vi "LvDataToMemory_PTR.vi"(8 "error in (no error)":errorcluster, 10 "Payload":variant, 11 "AddrQueueIn":refnum<queue>) -> (0 "error out":errorcluster, 1 "Supported Type?":bool, 2 "ByteArray":u8[](array[numeric]), 3 "AddrQueueOut":refnum<queue>)   [LabVIEW 2019, in "Memory Data Access.lvlib"]
uses:
  Memory Data Access.lvlib
  <vilib>/Utility/Data Type/Type Definitions/Data Type.ctl
  Global/Global.vi
  <vilib>/Utility/Data Type/NI_Data Type.lvlib
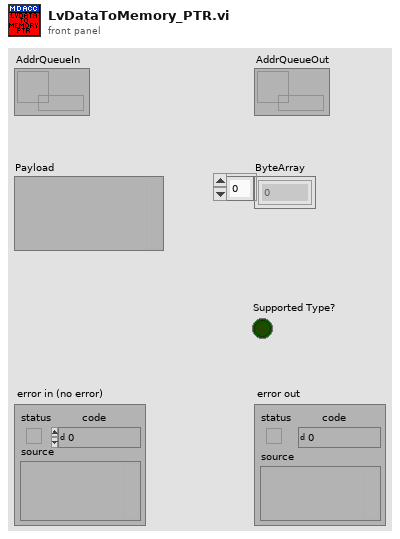
[diagram p1: front panel]
types:
  T1 = typedef "NI_Data Type.lvlib/Data Type.ctl" = enum8{"Invalid Type", "Void", "I8", "I16", "I32", "I64", "U8", "U16", "U32", "U64", "Single Float", "Double Float", "Extended Float", "Single Complex", "Double Complex", "Extended Complex", "Enum U8", "Enum U16", "Enum U32", "Enum U64", "Single Float With Unit", "Double Float With Unit", "Extended Float With Unit", "Single Complex with Unit", "Double Complex with Unit", "Extended Complex with Unit", "Boolean", "String", "Path", "Picture", "Tag", "Array", "Cluster", "Variant", "LV Variant", "Waveform", "Timestamp", "Digital Waveform", "Digital Data", "ExpressData", "Refnum", "External Data", "VI", "Poly VI", "LabVIEW Class Instance", "Fixed Point", "Set Collection", "Map Collection"}
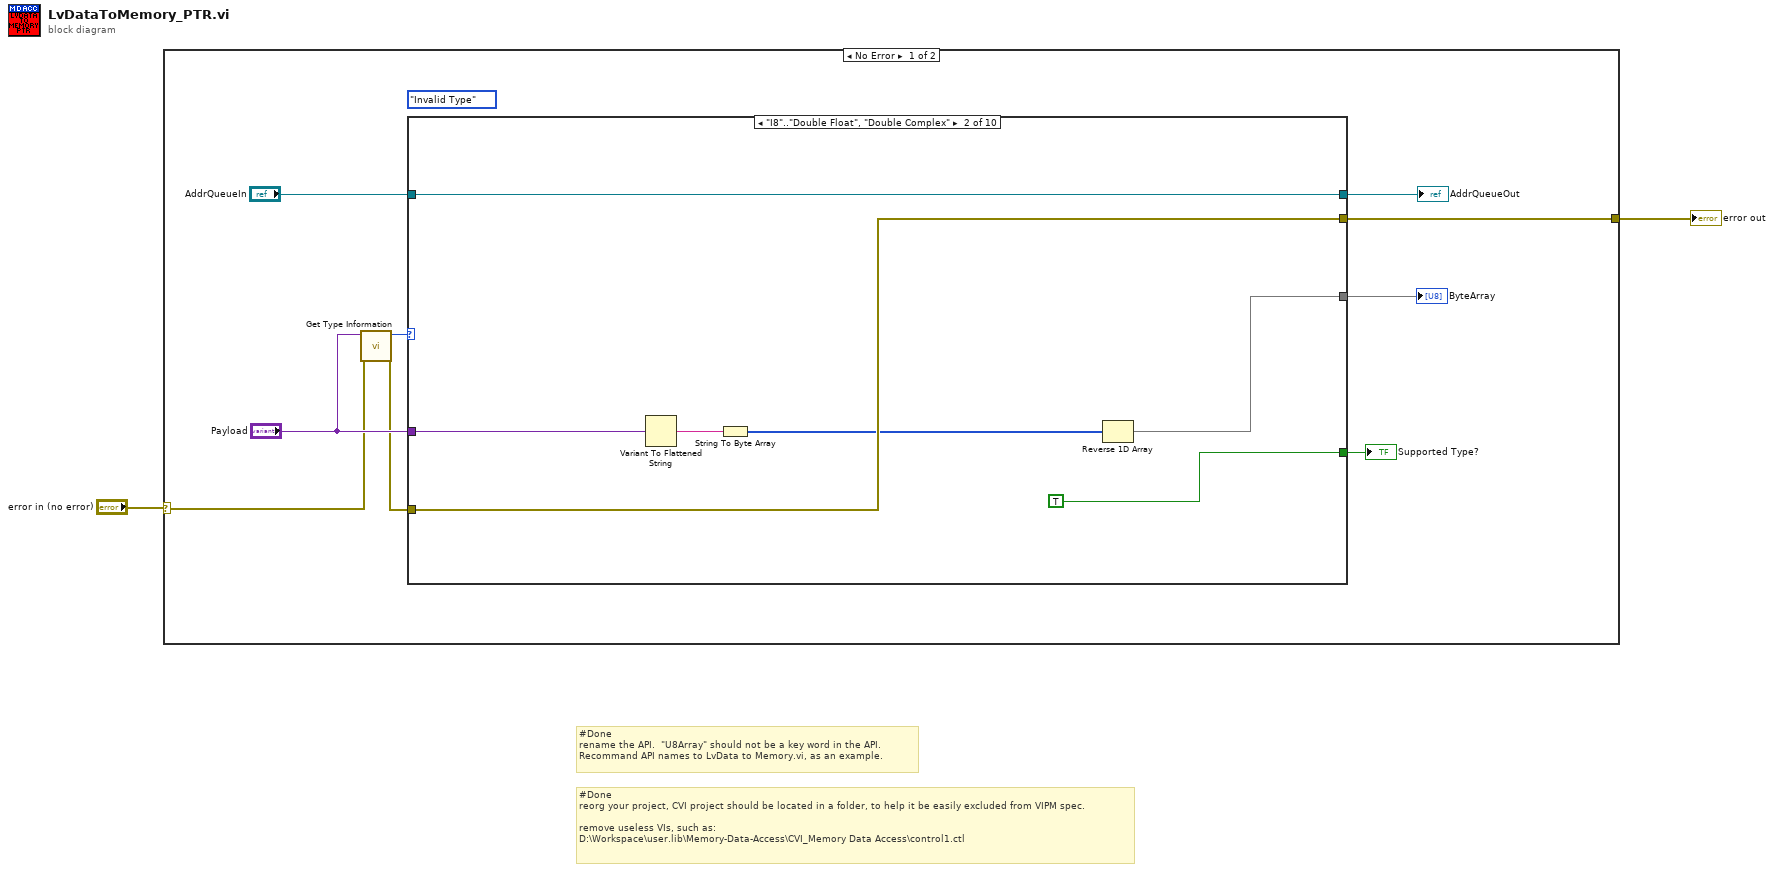
[diagram p0: block diagram]
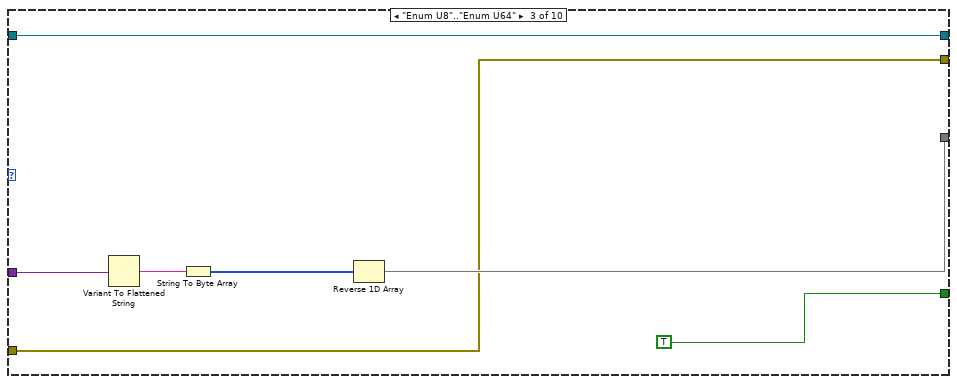
[diagram p3: hidden frame]
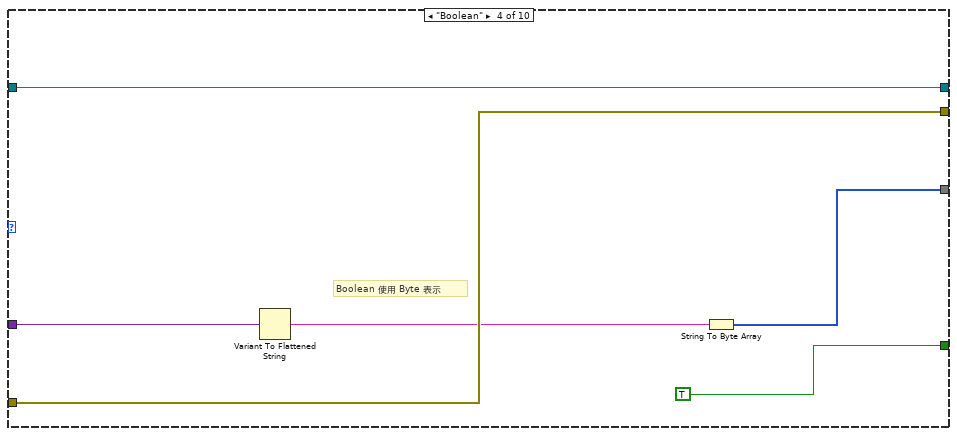
[diagram p4: hidden frame]
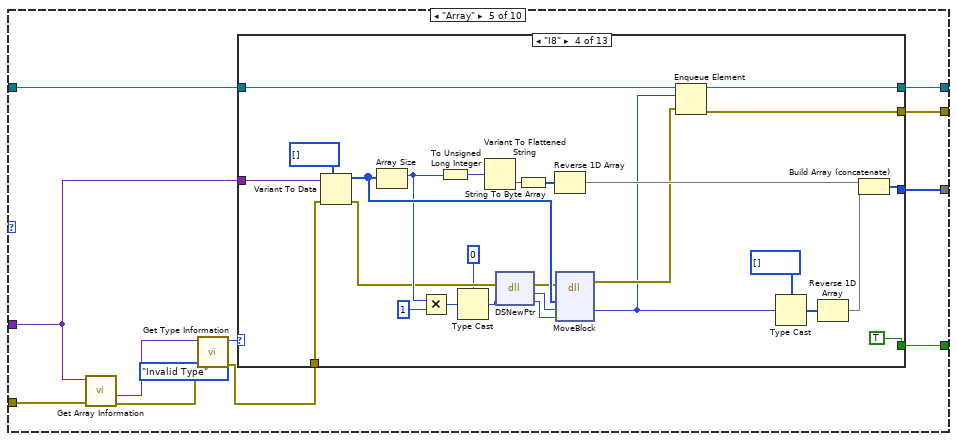
[diagram p5: hidden frame]
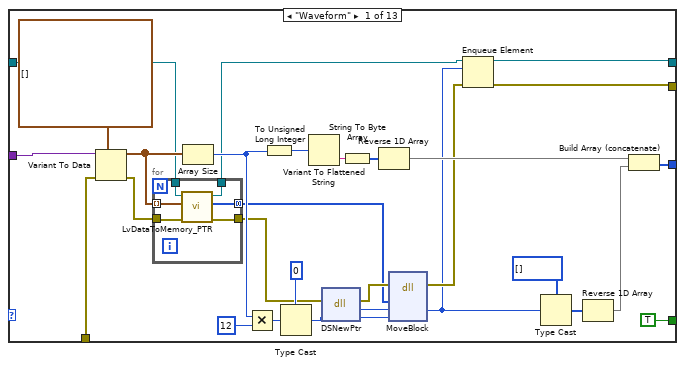
[diagram p6: hidden frame]
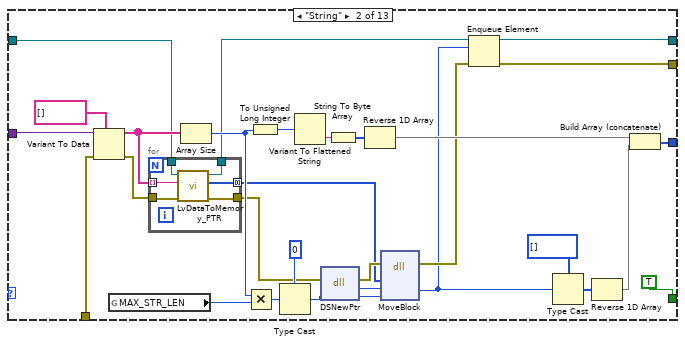
[diagram p7: hidden frame]
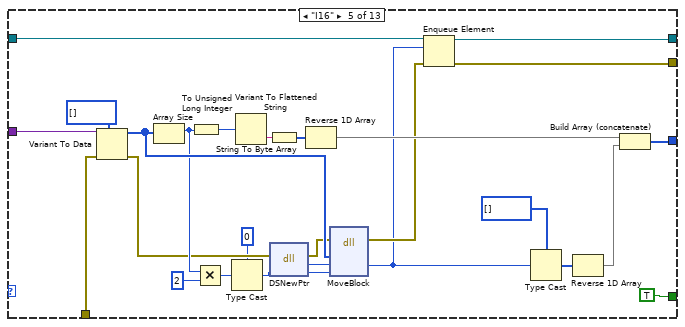
[diagram p9: hidden frame]
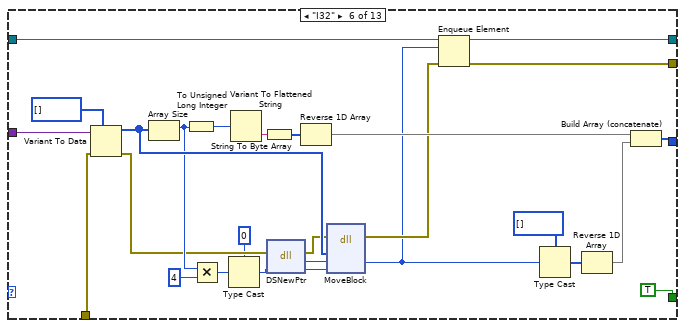
[diagram p10: hidden frame]
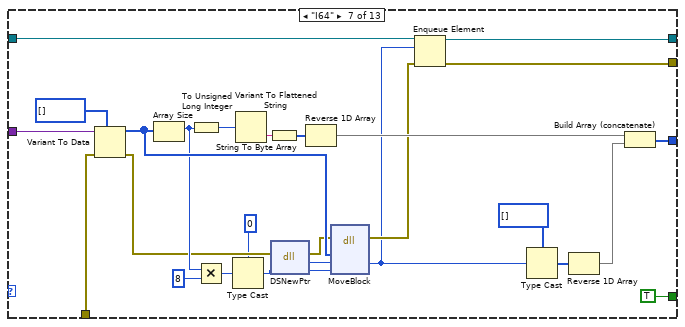
[diagram p11: hidden frame]
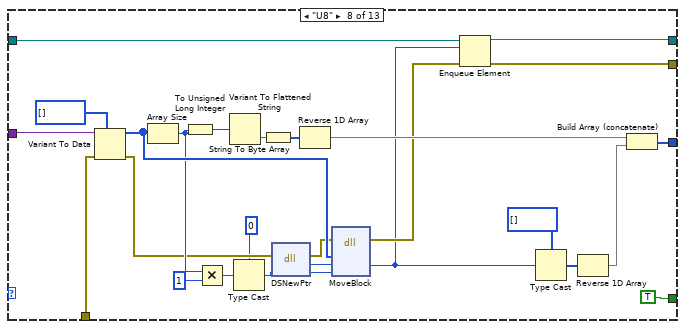
[diagram p12: hidden frame]
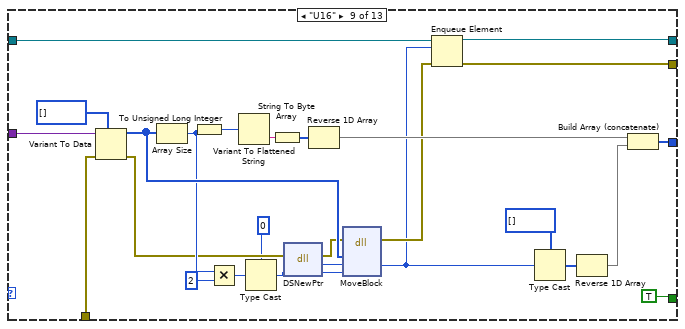
[diagram p13: hidden frame]
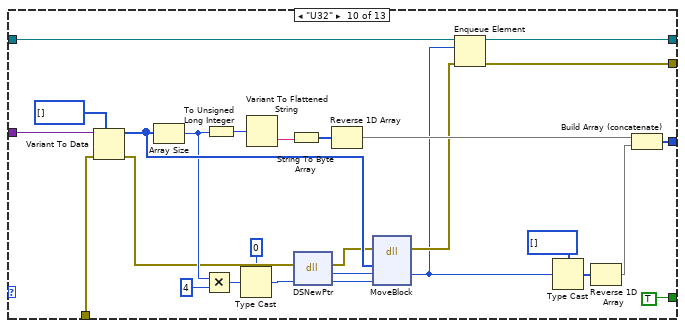
[diagram p14: hidden frame]
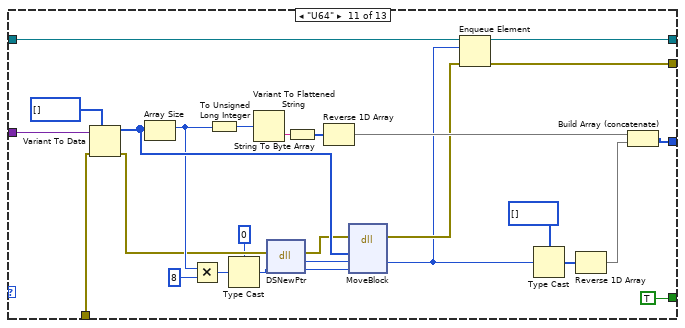
[diagram p15: hidden frame]
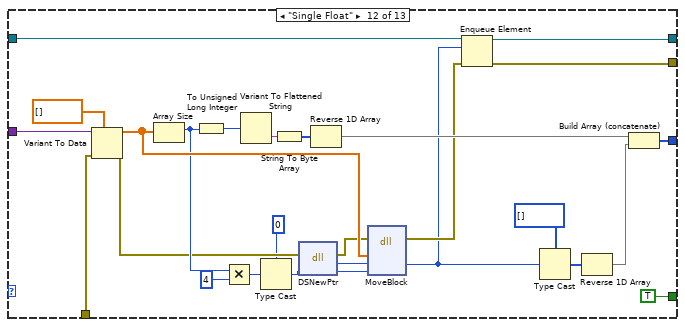
[diagram p16: hidden frame]
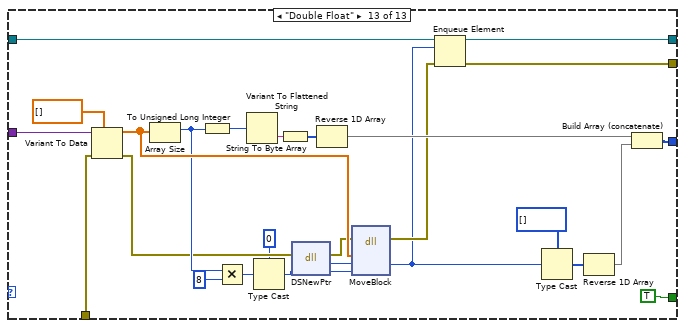
[diagram p17: hidden frame]
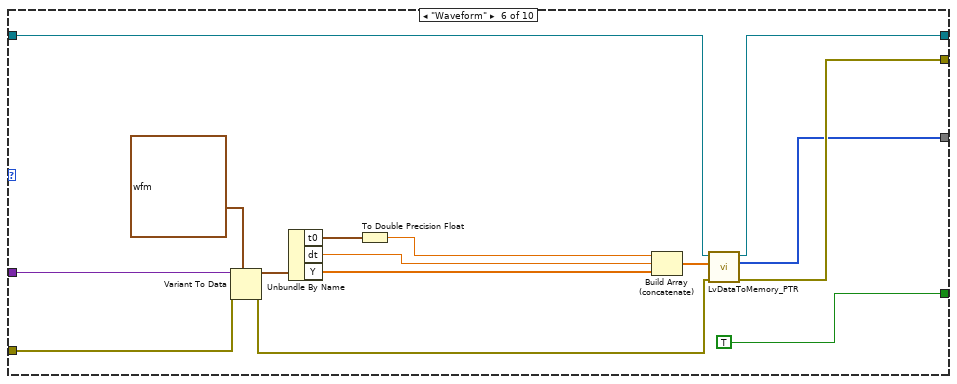
[diagram p18: hidden frame]
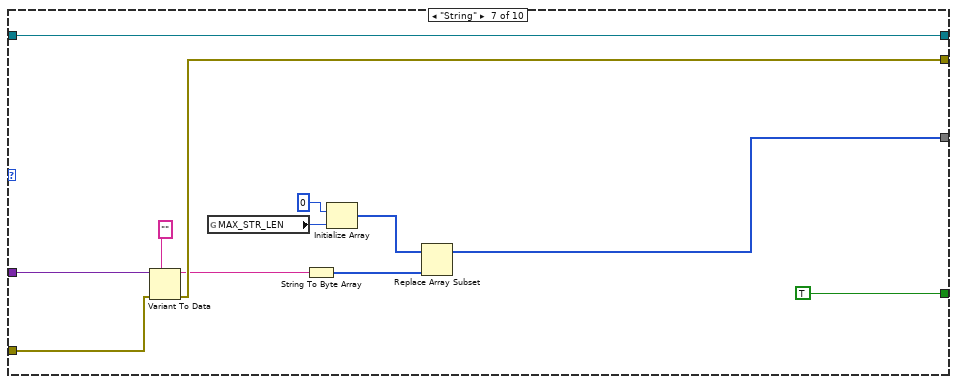
[diagram p19: hidden frame]
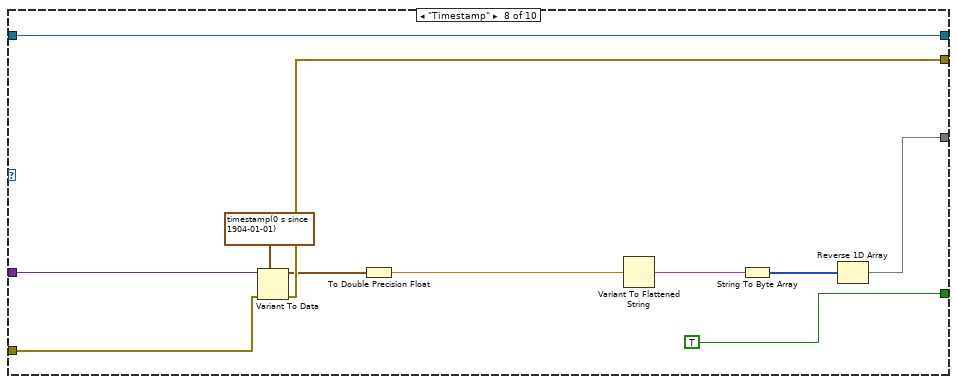
[diagram p20: hidden frame]
diagram:
  # "#Done\nreorg your project, CVI project should be located in a folder, to help it be easily excluded from VIPM spec.\n\nremove useless VIs, such as:\nD:\\Workspace\\user.lib\\Memory-Data-Access\\CVI_Memory Data Access\\control1.ctl"
  # "#Done\nrename the API.  \"U8Array\" should not be a key word in the API.\nRecommand API names to LvData to Memory.vi, as an example."
  n1 = case shown="No Error" "error in (no error)" {
    selector: "error in (no error)" -> [w3 w458]
    tunnel: [w11 w458] -> w2
    frame No Error {
      (unwired) Data_Type."Invalid Type" ("Type")
      n2 = call <vilib>:"Get Type Information.vi"("error in (no error)"=w3, "variant"="Payload") -> ("error out"=w6:errorcluster, "type"=w7:T1)  [unwired: 5 in, 3 out]
      n3 = case shown="\"I8\"..\"Double Float\", \"Double Complex\"" w7 {
        tunnel: w6 -> [w13 w20 w23 w33 w41 w395 w410 w421 w430 w442]
        tunnel: [w13 w20 w23 w33 w43 w392 w411 w422 w431 w443] -> w11
        tunnel: [_ w15 w24 w29 w44 w391 w413 w417 w433 w447] -> w10
        tunnel: "Payload" -> [_ w18 w26 w31 w42 w402 w414 w425 w434 w450]
        tunnel: [_ TRUE TRUE ("Supported Type?") TRUE w34 TRUE TRUE TRUE TRUE w445] -> w9
        tunnel: "AddrQueueIn" -> [w12 w14 w21 w28 w37 w390 w408 w416 w427 w441]
        tunnel: [w12 w14 w21 w28 w36 w389 w408 w416 w427 w440] -> w4
        frame "Invalid Type", Default {
        }
        frame "I8".."Double Float", "Double Complex" {
          n4 = Variant To Flattened String(Variant=w18) -> (data string=w17:string)  [unwired: 1 out]
          n5 = String To Byte Array(string=w17) -> (unsigned byte array=w16:u8[])
          n6 = Reverse 1D Array(array=w16) -> (reversed array=w15:u8[])
        }
        frame "Enum U8".."Enum U64" {
          n7 = Variant To Flattened String(Variant=w26) -> (data string=w27:string)  [unwired: 1 out]
          n8 = String To Byte Array(string=w27) -> (unsigned byte array=w25:u8[])
          n9 = Reverse 1D Array(array=w25) -> (reversed array=w24:u8[])
        }
        frame "Boolean" {
          # "Boolean 使用 Byte 表示"
          n10 = Variant To Flattened String(Variant=w31) -> (data string=w30:string)  [unwired: 1 out]
          n11 = String To Byte Array(string=w30) -> (unsigned byte array=w29:u8[])
        }
        frame "Array" {
          (unwired) Data_Type."Invalid Type" ("type")
          n12 = call <vilib>:"Get Array Information.vi"("error in (no error)"=w41, "variant"=w42) -> ("error out"=w35:errorcluster, "array element data type"=w39:variant)  [unwired: 6 in, 2 out]
          n13 = call <vilib>:"Get Type Information.vi"("error in (no error)"=w35, "variant"=w39) -> ("error out"=w38:errorcluster, "type"=w40:T1)  [unwired: 5 in, 3 out]
          n14 = case shown="\"I8\"" w40 {
            tunnel: [w55 w94 _ w125 w153 w180 w207 w233 w260 w287 w314 w341 w368] -> w44
            tunnel: w42 -> [w54 w95 _ w127 w154 w181 w208 w235 w262 w290 w316 w343 w370]
            tunnel: w38 -> [w53 w93 w117 w126 w152 w179 w206 w234 w261 w289 w315 w342 w369]
            tunnel: [w48 w85 w117 w121 w149 w175 w201 w228 w256 w284 w310 w337 w365] -> w43
            tunnel: w37 -> [w47 w84 w118 w124 w151 w178 w205 w232 w259 w286 w313 w340 w367]
            tunnel: [w52 w87 w118 w123 w150 w177 w204 w231 w258 w282 w312 w339 w364] -> w36
            tunnel: [TRUE ("Supported Type?") TRUE ("Supported Type?") _ TRUE ("Supported Type?") TRUE ("Supported Type?") TRUE ("Supported Type?") TRUE ("Supported Type?") TRUE ("Supported Type?") TRUE ("Supported Type?") TRUE ("Supported Type?") TRUE ("Supported Type?") TRUE ("Supported Type?") TRUE ("Supported Type?")] -> w34
            frame "Waveform" {
              n15 = Variant To Data(error in=w53, type=waveform(dbl)[] [], Variant=w54) -> (data=w59:waveform(dbl)[], error out=w58:errorcluster)
              n16 = for {
                tunnel: w59 -> [w80] mode=indexing
                tunnel: w58 -> [w79]
                tunnel: [w78] -> w56 mode=concatenating
                tunnel: [w77] -> w57
                tunnel: w47 -> [w76]
                tunnel: [w75] -> w46
                n17 = call "LvDataToMemory_PTR.vi"("error in (no error)"=w79, "Payload"=w80, "AddrQueueIn"=w76) -> ("error out"=w77:errorcluster, "ByteArray"=w78:u8[], "AddrQueueOut"=w75:refnum<queue>)  [unwired: 5 in, 1 out]
              }
              n18 = Array Size(array=w59) -> (size(s)=w70:i32)
              n19 = Multiply(x=w70, y=12) -> (x*y=w71:i32)
              n20 = To Unsigned Long Integer(number=w70) -> (unsigned 32bit integer=w67:u32)
              n21 = Type Cast(type=u32 0, x=w71) -> (*(type *) &x=w72:u32)
              n22 = Variant To Flattened String(Variant=w67) -> (data string=w66:string)  [unwired: 1 out]
              n23 = dll-call lib="LabVIEW" fn="DSNewPtr"(error in=w57, "size"=w72) -> (error out=w63:errorcluster, "return type"=w73:u64, "size"=w74:u32)  [unwired: 2 in, 1 out]
              n24 = String To Byte Array(string=w66) -> (unsigned byte array=w68:u8[])
              n25 = Reverse 1D Array(array=w68) -> (reversed array=w69:u8[])
              n26 = dll-call lib="LabVIEW" fn="MoveBlock"(error in=w63, "PointerSRC"=w56, "PointerDEST"=w73, "size"=w74) -> (error out=w50:errorcluster, "PointerDEST"=w49:u64)  [unwired: 5 in, 1 out]
              n27 = Enqueue Element(queue=w46, element=w49, error in (no error)=w50) -> (queue out=w52:refnum<queue>, error out=w48:errorcluster)  [unwired: 1 in, 1 out]
              n28 = Type Cast(type=u8[] [], x=w49) -> (*(type *) &x=w65:u8[])
              n29 = Reverse 1D Array(array=w65) -> (reversed array=w64:u8[])
              n30 = Build Array (concatenate)(w69, w64) -> (w55:u8[])
            }
            frame "String" {
              n31 = Variant To Data(error in=w93, type=string[] [], Variant=w95) -> (data=w92:string[], error out=w91:errorcluster)
              n32 = global read "Global.vi" "MAX_STR_LEN"() -> (w88:u32)
              n33 = for {
                tunnel: w92 -> [w116] mode=indexing
                tunnel: w91 -> [w115]
                tunnel: [w114] -> w89 mode=concatenating
                tunnel: [w113] -> w90
                tunnel: w84 -> [w112]
                tunnel: [w111] -> w82
                n34 = call "LvDataToMemory_PTR.vi"("error in (no error)"=w115, "Payload"=w116, "AddrQueueIn"=w112) -> ("error out"=w113:errorcluster, "ByteArray"=w114:u8[], "AddrQueueOut"=w111:refnum<queue>)  [unwired: 5 in, 1 out]
              }
              n35 = Array Size(array=w92) -> (size(s)=w106:i32)
              n36 = Multiply(x=w106, y=w88) -> (x*y=w107:u32)
              n37 = To Unsigned Long Integer(number=w106) -> (unsigned 32bit integer=w103:u32)
              n38 = Type Cast(type=u32 0, x=w107) -> (*(type *) &x=w108:u32)
              n39 = Variant To Flattened String(Variant=w103) -> (data string=w102:string)  [unwired: 1 out]
              n40 = dll-call lib="LabVIEW" fn="DSNewPtr"(error in=w90, "size"=w108) -> (error out=w99:errorcluster, "return type"=w109:u64, "size"=w110:u32)  [unwired: 2 in, 1 out]
              n41 = String To Byte Array(string=w102) -> (unsigned byte array=w104:u8[])
              n42 = Reverse 1D Array(array=w104) -> (reversed array=w105:u8[])
              n43 = dll-call lib="LabVIEW" fn="MoveBlock"(error in=w99, "PointerSRC"=w89, "PointerDEST"=w109, "size"=w110) -> (error out=w86:errorcluster, "PointerDEST"=w83:u64)  [unwired: 5 in, 1 out]
              n44 = Enqueue Element(queue=w82, element=w83, error in (no error)=w86) -> (queue out=w87:refnum<queue>, error out=w85:errorcluster)  [unwired: 1 in, 1 out]
              n45 = Type Cast(type=u8[] [], x=w83) -> (*(type *) &x=w101:u8[])
              n46 = Reverse 1D Array(array=w101) -> (reversed array=w100:u8[])
              n47 = Build Array (concatenate)(w105, w100) -> (w94:u8[])
            }
            frame "Invalid Type", Default {
            }
            frame "I8" {
              n48 = Variant To Data(error in=w126, type=i8[] [], Variant=w127) -> (data=w143:i8[], error out=w135:errorcluster)
              n49 = Array Size(array=w143) -> (size(s)=w140:i32)
              n50 = Multiply(x=w140, y=1) -> (x*y=w141:i32)
              n51 = To Unsigned Long Integer(number=w140) -> (unsigned 32bit integer=w137:u32)
              n52 = Type Cast(type=u32 0, x=w141) -> (*(type *) &x=w142:u32)
              n53 = Variant To Flattened String(Variant=w137) -> (data string=w136:string)  [unwired: 1 out]
              n54 = dll-call lib="LabVIEW" fn="DSNewPtr"(error in=w135, "size"=w142) -> (error out=w132:errorcluster, "return type"=w144:u64, "size"=w145:u32)  [unwired: 2 in, 1 out]
              n55 = String To Byte Array(string=w136) -> (unsigned byte array=w138:u8[])
              n56 = Reverse 1D Array(array=w138) -> (reversed array=w139:u8[])
              n57 = dll-call lib="LabVIEW" fn="MoveBlock"(error in=w132, "PointerSRC"=w143, "PointerDEST"=w144, "size"=w145) -> (error out=w122:errorcluster, "PointerDEST"=w120:u64)  [unwired: 5 in, 1 out]
              n58 = Enqueue Element(queue=w124, element=w120, error in (no error)=w122) -> (queue out=w123:refnum<queue>, error out=w121:errorcluster)  [unwired: 1 in, 1 out]
              n59 = Type Cast(type=u8[] [], x=w120) -> (*(type *) &x=w134:u8[])
              n60 = Reverse 1D Array(array=w134) -> (reversed array=w133:u8[])
              n61 = Build Array (concatenate)(w139, w133) -> (w125:u8[])
            }
            frame "I16" {
              n62 = Variant To Data(error in=w152, type=i16[] [], Variant=w154) -> (data=w170:i16[], error out=w162:errorcluster)
              n63 = Array Size(array=w170) -> (size(s)=w167:i32)
              n64 = To Unsigned Long Integer(number=w167) -> (unsigned 32bit integer=w164:u32)
              n65 = Multiply(x=w167, y=2) -> (x*y=w168:i32)
              n66 = Type Cast(type=u32 0, x=w168) -> (*(type *) &x=w169:u32)
              n67 = Variant To Flattened String(Variant=w164) -> (data string=w163:string)  [unwired: 1 out]
              n68 = String To Byte Array(string=w163) -> (unsigned byte array=w165:u8[])
              n69 = dll-call lib="LabVIEW" fn="DSNewPtr"(error in=w162, "size"=w169) -> (error out=w159:errorcluster, "return type"=w171:u64, "size"=w172:u32)  [unwired: 2 in, 1 out]
              n70 = Reverse 1D Array(array=w165) -> (reversed array=w166:u8[])
              n71 = dll-call lib="LabVIEW" fn="MoveBlock"(error in=w159, "PointerSRC"=w170, "PointerDEST"=w171, "size"=w172) -> (error out=w148:errorcluster, "PointerDEST"=w147:u64)  [unwired: 5 in, 1 out]
              n72 = Enqueue Element(queue=w151, element=w147, error in (no error)=w148) -> (queue out=w150:refnum<queue>, error out=w149:errorcluster)  [unwired: 1 in, 1 out]
              n73 = Type Cast(type=u8[] [], x=w147) -> (*(type *) &x=w161:u8[])
              n74 = Reverse 1D Array(array=w161) -> (reversed array=w160:u8[])
              n75 = Build Array (concatenate)(w166, w160) -> (w153:u8[])
            }
            frame "I32" {
              n76 = Variant To Data(error in=w179, type=i32[] [], Variant=w181) -> (data=w197:i32[], error out=w189:errorcluster)
              n77 = Array Size(array=w197) -> (size(s)=w194:i32)
              n78 = To Unsigned Long Integer(number=w194) -> (unsigned 32bit integer=w191:u32)
              n79 = Multiply(x=w194, y=4) -> (x*y=w195:i32)
              n80 = Type Cast(type=u32 0, x=w195) -> (*(type *) &x=w196:u32)
              n81 = Variant To Flattened String(Variant=w191) -> (data string=w190:string)  [unwired: 1 out]
              n82 = String To Byte Array(string=w190) -> (unsigned byte array=w192:u8[])
              n83 = dll-call lib="LabVIEW" fn="DSNewPtr"(error in=w189, "size"=w196) -> (error out=w186:errorcluster, "return type"=w198:u64, "size"=w199:u32)  [unwired: 2 in, 1 out]
              n84 = Reverse 1D Array(array=w192) -> (reversed array=w193:u8[])
              n85 = dll-call lib="LabVIEW" fn="MoveBlock"(error in=w186, "PointerSRC"=w197, "PointerDEST"=w198, "size"=w199) -> (error out=w176:errorcluster, "PointerDEST"=w174:u64)  [unwired: 5 in, 1 out]
              n86 = Enqueue Element(queue=w178, element=w174, error in (no error)=w176) -> (queue out=w177:refnum<queue>, error out=w175:errorcluster)  [unwired: 1 in, 1 out]
              n87 = Type Cast(type=u8[] [], x=w174) -> (*(type *) &x=w188:u8[])
              n88 = Reverse 1D Array(array=w188) -> (reversed array=w187:u8[])
              n89 = Build Array (concatenate)(w193, w187) -> (w180:u8[])
            }
            frame "I64" {
              n90 = Variant To Data(error in=w206, type=i64[] [], Variant=w208) -> (data=w224:i64[], error out=w216:errorcluster)
              n91 = Array Size(array=w224) -> (size(s)=w221:i32)
              n92 = To Unsigned Long Integer(number=w221) -> (unsigned 32bit integer=w218:u32)
              n93 = Multiply(x=w221, y=8) -> (x*y=w222:i32)
              n94 = Type Cast(type=u32 0, x=w222) -> (*(type *) &x=w223:u32)
              n95 = Variant To Flattened String(Variant=w218) -> (data string=w217:string)  [unwired: 1 out]
              n96 = String To Byte Array(string=w217) -> (unsigned byte array=w219:u8[])
              n97 = dll-call lib="LabVIEW" fn="DSNewPtr"(error in=w216, "size"=w223) -> (error out=w213:errorcluster, "return type"=w225:u64, "size"=w226:u32)  [unwired: 2 in, 1 out]
              n98 = Reverse 1D Array(array=w219) -> (reversed array=w220:u8[])
              n99 = dll-call lib="LabVIEW" fn="MoveBlock"(error in=w213, "PointerSRC"=w224, "PointerDEST"=w225, "size"=w226) -> (error out=w203:errorcluster, "PointerDEST"=w202:u64)  [unwired: 5 in, 1 out]
              n100 = Enqueue Element(queue=w205, element=w202, error in (no error)=w203) -> (queue out=w204:refnum<queue>, error out=w201:errorcluster)  [unwired: 1 in, 1 out]
              n101 = Type Cast(type=u8[] [], x=w202) -> (*(type *) &x=w215:u8[])
              n102 = Reverse 1D Array(array=w215) -> (reversed array=w214:u8[])
              n103 = Build Array (concatenate)(w220, w214) -> (w207:u8[])
            }
            frame "U8" {
              n104 = Variant To Data(error in=w234, type=u8[] [], Variant=w235) -> (data=w251:u8[], error out=w243:errorcluster)
              n105 = Array Size(array=w251) -> (size(s)=w248:i32)
              n106 = To Unsigned Long Integer(number=w248) -> (unsigned 32bit integer=w245:u32)
              n107 = Multiply(x=w248, y=1) -> (x*y=w249:i32)
              n108 = Variant To Flattened String(Variant=w245) -> (data string=w244:string)  [unwired: 1 out]
              n109 = Type Cast(type=u32 0, x=w249) -> (*(type *) &x=w250:u32)
              n110 = String To Byte Array(string=w244) -> (unsigned byte array=w246:u8[])
              n111 = dll-call lib="LabVIEW" fn="DSNewPtr"(error in=w243, "size"=w250) -> (error out=w240:errorcluster, "return type"=w252:u64, "size"=w253:u32)  [unwired: 2 in, 1 out]
              n112 = Reverse 1D Array(array=w246) -> (reversed array=w247:u8[])
              n113 = dll-call lib="LabVIEW" fn="MoveBlock"(error in=w240, "PointerSRC"=w251, "PointerDEST"=w252, "size"=w253) -> (error out=w230:errorcluster, "PointerDEST"=w229:u64)  [unwired: 5 in, 1 out]
              n114 = Enqueue Element(queue=w232, element=w229, error in (no error)=w230) -> (queue out=w231:refnum<queue>, error out=w228:errorcluster)  [unwired: 1 in, 1 out]
              n115 = Type Cast(type=u8[] [], x=w229) -> (*(type *) &x=w242:u8[])
              n116 = Reverse 1D Array(array=w242) -> (reversed array=w241:u8[])
              n117 = Build Array (concatenate)(w247, w241) -> (w233:u8[])
            }
            frame "U16" {
              n118 = Variant To Data(error in=w261, type=u16[] [], Variant=w262) -> (data=w278:u16[], error out=w270:errorcluster)
              n119 = Array Size(array=w278) -> (size(s)=w275:i32)
              n120 = To Unsigned Long Integer(number=w275) -> (unsigned 32bit integer=w272:u32)
              n121 = Multiply(x=w275, y=2) -> (x*y=w276:i32)
              n122 = Variant To Flattened String(Variant=w272) -> (data string=w271:string)  [unwired: 1 out]
              n123 = Type Cast(type=u32 0, x=w276) -> (*(type *) &x=w277:u32)
              n124 = String To Byte Array(string=w271) -> (unsigned byte array=w273:u8[])
              n125 = dll-call lib="LabVIEW" fn="DSNewPtr"(error in=w270, "size"=w277) -> (error out=w267:errorcluster, "return type"=w279:u64, "size"=w280:u32)  [unwired: 2 in, 1 out]
              n126 = Reverse 1D Array(array=w273) -> (reversed array=w274:u8[])
              n127 = dll-call lib="LabVIEW" fn="MoveBlock"(error in=w267, "PointerSRC"=w278, "PointerDEST"=w279, "size"=w280) -> (error out=w257:errorcluster, "PointerDEST"=w255:u64)  [unwired: 5 in, 1 out]
              n128 = Enqueue Element(queue=w259, element=w255, error in (no error)=w257) -> (queue out=w258:refnum<queue>, error out=w256:errorcluster)  [unwired: 1 in, 1 out]
              n129 = Type Cast(type=u8[] [], x=w255) -> (*(type *) &x=w269:u8[])
              n130 = Reverse 1D Array(array=w269) -> (reversed array=w268:u8[])
              n131 = Build Array (concatenate)(w274, w268) -> (w260:u8[])
            }
            frame "U32" {
              n132 = Variant To Data(error in=w289, type=u32[] [], Variant=w290) -> (data=w305:u32[], error out=w297:errorcluster)
              n133 = Array Size(array=w305) -> (size(s)=w302:i32)
              n134 = Multiply(x=w302, y=4) -> (x*y=w303:i32)
              n135 = To Unsigned Long Integer(number=w302) -> (unsigned 32bit integer=w299:u32)
              n136 = Type Cast(type=u32 0, x=w303) -> (*(type *) &x=w304:u32)
              n137 = Variant To Flattened String(Variant=w299) -> (data string=w298:string)  [unwired: 1 out]
              n138 = String To Byte Array(string=w298) -> (unsigned byte array=w300:u8[])
              n139 = dll-call lib="LabVIEW" fn="DSNewPtr"(error in=w297, "size"=w304) -> (error out=w294:errorcluster, "return type"=w306:u64, "size"=w307:u32)  [unwired: 2 in, 1 out]
              n140 = Reverse 1D Array(array=w300) -> (reversed array=w301:u8[])
              n141 = dll-call lib="LabVIEW" fn="MoveBlock"(error in=w294, "PointerSRC"=w305, "PointerDEST"=w306, "size"=w307) -> (error out=w285:errorcluster, "PointerDEST"=w283:u64)  [unwired: 5 in, 1 out]
              n142 = Enqueue Element(queue=w286, element=w283, error in (no error)=w285) -> (queue out=w282:refnum<queue>, error out=w284:errorcluster)  [unwired: 1 in, 1 out]
              n143 = Type Cast(type=u8[] [], x=w283) -> (*(type *) &x=w296:u8[])
              n144 = Reverse 1D Array(array=w296) -> (reversed array=w295:u8[])
              n145 = Build Array (concatenate)(w301, w295) -> (w287:u8[])
            }
            frame "U64" {
              n146 = Variant To Data(error in=w315, type=u64[] [], Variant=w316) -> (data=w332:u64[], error out=w324:errorcluster)
              n147 = Array Size(array=w332) -> (size(s)=w329:i32)
              n148 = Multiply(x=w329, y=8) -> (x*y=w330:i32)
              n149 = To Unsigned Long Integer(number=w329) -> (unsigned 32bit integer=w326:u32)
              n150 = Type Cast(type=u32 0, x=w330) -> (*(type *) &x=w331:u32)
              n151 = Variant To Flattened String(Variant=w326) -> (data string=w325:string)  [unwired: 1 out]
              n152 = dll-call lib="LabVIEW" fn="DSNewPtr"(error in=w324, "size"=w331) -> (error out=w321:errorcluster, "return type"=w333:u64, "size"=w334:u32)  [unwired: 2 in, 1 out]
              n153 = String To Byte Array(string=w325) -> (unsigned byte array=w327:u8[])
              n154 = Reverse 1D Array(array=w327) -> (reversed array=w328:u8[])
              n155 = dll-call lib="LabVIEW" fn="MoveBlock"(error in=w321, "PointerSRC"=w332, "PointerDEST"=w333, "size"=w334) -> (error out=w311:errorcluster, "PointerDEST"=w309:u64)  [unwired: 5 in, 1 out]
              n156 = Enqueue Element(queue=w313, element=w309, error in (no error)=w311) -> (queue out=w312:refnum<queue>, error out=w310:errorcluster)  [unwired: 1 in, 1 out]
              n157 = Type Cast(type=u8[] [], x=w309) -> (*(type *) &x=w323:u8[])
              n158 = Reverse 1D Array(array=w323) -> (reversed array=w322:u8[])
              n159 = Build Array (concatenate)(w328, w322) -> (w314:u8[])
            }
            frame "Single Float" {
              n160 = Variant To Data(error in=w342, type=sgl[] [], Variant=w343) -> (data=w359:sgl[], error out=w351:errorcluster)
              n161 = Array Size(array=w359) -> (size(s)=w356:i32)
              n162 = To Unsigned Long Integer(number=w356) -> (unsigned 32bit integer=w353:u32)
              n163 = Multiply(x=w356, y=4) -> (x*y=w357:i32)
              n164 = Variant To Flattened String(Variant=w353) -> (data string=w352:string)  [unwired: 1 out]
              n165 = Type Cast(type=u32 0, x=w357) -> (*(type *) &x=w358:u32)
              n166 = String To Byte Array(string=w352) -> (unsigned byte array=w354:u8[])
              n167 = dll-call lib="LabVIEW" fn="DSNewPtr"(error in=w351, "size"=w358) -> (error out=w348:errorcluster, "return type"=w360:u64, "size"=w361:u32)  [unwired: 2 in, 1 out]
              n168 = Reverse 1D Array(array=w354) -> (reversed array=w355:u8[])
              n169 = dll-call lib="LabVIEW" fn="MoveBlock"(error in=w348, "PointerSRC"=w359, "PointerDEST"=w360, "size"=w361) -> (error out=w338:errorcluster, "PointerDEST"=w336:u64)  [unwired: 5 in, 1 out]
              n170 = Enqueue Element(queue=w340, element=w336, error in (no error)=w338) -> (queue out=w339:refnum<queue>, error out=w337:errorcluster)  [unwired: 1 in, 1 out]
              n171 = Type Cast(type=u8[] [], x=w336) -> (*(type *) &x=w350:u8[])
              n172 = Reverse 1D Array(array=w350) -> (reversed array=w349:u8[])
              n173 = Build Array (concatenate)(w355, w349) -> (w341:u8[])
            }
            frame "Double Float" {
              n174 = Variant To Data(error in=w369, type=dbl[] [], Variant=w370) -> (data=w386:dbl[], error out=w378:errorcluster)
              n175 = Array Size(array=w386) -> (size(s)=w383:i32)
              n176 = To Unsigned Long Integer(number=w383) -> (unsigned 32bit integer=w380:u32)
              n177 = Multiply(x=w383, y=8) -> (x*y=w384:i32)
              n178 = Variant To Flattened String(Variant=w380) -> (data string=w379:string)  [unwired: 1 out]
              n179 = Type Cast(type=u32 0, x=w384) -> (*(type *) &x=w385:u32)
              n180 = String To Byte Array(string=w379) -> (unsigned byte array=w381:u8[])
              n181 = dll-call lib="LabVIEW" fn="DSNewPtr"(error in=w378, "size"=w385) -> (error out=w375:errorcluster, "return type"=w387:u64, "size"=w388:u32)  [unwired: 2 in, 1 out]
              n182 = Reverse 1D Array(array=w381) -> (reversed array=w382:u8[])
              n183 = dll-call lib="LabVIEW" fn="MoveBlock"(error in=w375, "PointerSRC"=w386, "PointerDEST"=w387, "size"=w388) -> (error out=w366:errorcluster, "PointerDEST"=w363:u64)  [unwired: 5 in, 1 out]
              n184 = Enqueue Element(queue=w367, element=w363, error in (no error)=w366) -> (queue out=w364:refnum<queue>, error out=w365:errorcluster)  [unwired: 1 in, 1 out]
              n185 = Type Cast(type=u8[] [], x=w363) -> (*(type *) &x=w377:u8[])
              n186 = Reverse 1D Array(array=w377) -> (reversed array=w376:u8[])
              n187 = Build Array (concatenate)(w382, w376) -> (w368:u8[])
            }
          }
        }
        frame "Waveform" {
          n188 = Variant To Data(error in=w395, type=waveform(dbl) {"t0"=timestamp(0 s since 1904-01-01), "dt"=1.0, "Y"=[]} ("Waveform"), Variant=w402) -> (data=w400:waveform(dbl), error out=w393:errorcluster)
          n189 = Unbundle By Name(w400) -> ("t0"=w398:timestamp, "dt"=w396:dbl, "Y"=w399:dbl[])
          n190 = To Double Precision Float(number=w398) -> (double precision float=w397:dbl)
          n191 = Build Array (concatenate)(w397, w396, w399) -> (w394:dbl[])
          n192 = call "LvDataToMemory_PTR.vi"("error in (no error)"=w393, "Payload"=w394, "AddrQueueIn"=w390) -> ("error out"=w392:errorcluster, "ByteArray"=w391:u8[], "AddrQueueOut"=w389:refnum<queue>)  [unwired: 5 in, 1 out]
        }
        frame "String" {
          n193 = Variant To Data(error in=w410, type="" ("Waveform"), Variant=w414) -> (data=w409:string, error out=w411:errorcluster)
          n194 = global read "Global.vi" "MAX_STR_LEN"() -> (w404:u32)
          n195 = String To Byte Array(string=w409) -> (unsigned byte array=w405:u8[])
          n196 = Initialize Array(u8 0 ("*(type *) &x"), w404) -> (w406:u8[])
          n197 = Replace Array Subset(array=w406, new element=w405) -> (w413:u8[])  [unwired: 1 in]
        }
        frame "Timestamp" {
          n198 = Variant To Data(error in=w421, type=timestamp(0 s since 1904-01-01) ("Waveform"), Variant=w425) -> (data=w420:timestamp, error out=w422:errorcluster)
          n199 = To Double Precision Float(number=w420) -> (double precision float=w419:dbl)
          n200 = Variant To Flattened String(Variant=w419) -> (data string=w424:string)  [unwired: 1 out]
          n201 = String To Byte Array(string=w424) -> (unsigned byte array=w418:u8[])
          n202 = Reverse 1D Array(array=w418) -> (reversed array=w417:u8[])
        }
        frame "Path" {
          n203 = Variant To Data(error in=w430, type=path "" ("Waveform"), Variant=w434) -> (data=w429:path, error out=w431:errorcluster)
          n204 = Path To String(path=w429) -> (string=w428:string)
          n205 = disable-structure shown="Enabled" {
            disable-tunnel: [w437 w438] -> w433
            disable-tunnel: w428 -> [w436 w439]
            frame Disabled {
              n206 = Variant To Flattened String(Variant=w436) -> (data string=w437:string)  [unwired: 1 out]
            }
            frame Enabled {
              n207 = String To Byte Array(string=w439) -> (unsigned byte array=w438:u8[])
            }
          }
        }
        frame "Cluster" {
          n208 = call <userlib>:"Cluster to Array of VData__ogtk.vi"("error in (no error)"=w442, "Cluster"=w450) -> ("error out"=w444:errorcluster, "Array of VData"=w449:variant[])  [unwired: 8 in]
          n209 = for {
            tunnel: w449 -> [w457] mode=indexing
            tunnel: [w456] -> w448 mode=concatenating
            tunnel: [w455] -> w446 mode=indexing
            shift-right: [w453] -> w443
            shift-left: w444 -> [w454]
            tunnel: w441 -> [w452]
            tunnel: [w451] -> w440
            n210 = call "LvDataToMemory_PTR.vi"("error in (no error)"=w454, "Payload"=w457, "AddrQueueIn"=w452) -> ("error out"=w453:errorcluster, "Supported Type?"=w455:bool, "ByteArray"=w456:u8[], "AddrQueueOut"=w451:refnum<queue>)  [unwired: 5 in]
          }
          n211 = Build Array (concatenate)(w448) -> (w447:u8[])
          n212 = And Array Elements(Boolean array=w446) -> (logical AND=w445:bool)
        }
      }
      "ByteArray" <- w10
      "Supported Type?" <- w9
      "AddrQueueOut" <- w4
    }
    frame Error {
    }
  }
  "error out" <- w2
